vi "DMM User Interface.vi"() -> ()   [LabVIEW 2023, in "GUI.lvlib" / "Diagnostic.lvlib"]
uses:
  Diagnostic.lvlib
  <instrlib>/niDMM/nidmm.llb/niDMM Resolution in Digits.ctl
  <instrlib>/niDMM/nidmm.llb/niDMM Function.ctl
panel:
  in  "Stop":bool caption="Blank"
  in  "Apply":bool caption="Blank"
  in  "DMM Operation":T1(tab)
  in  "DMM":refnum<k15>="PXI2Slot6"
  out "Measured Value":dbl=1e-06 caption="Absolute Resolution (1E-6)" format="%.4f"
  in  "Range":dbl=-1.0
  in  "Resolution in Digits":T2=5.5 items=["3 1/2"=3.5, "4 1/2"=4.5, "5 1/2"=5.5, "6 1/2"=6.5, "7 1/2"=7.5]
  in  "Measurement Function (DC Volts)":T3=enum."Diode" caption="Measurement Function"
  # "Digital MultiMeter"
  # "Operation:"
  # "Self Test is Enabled by selecting\n            this opeartion"
  # "DMM Close Operation will be executing \nby selecting this opeartion"
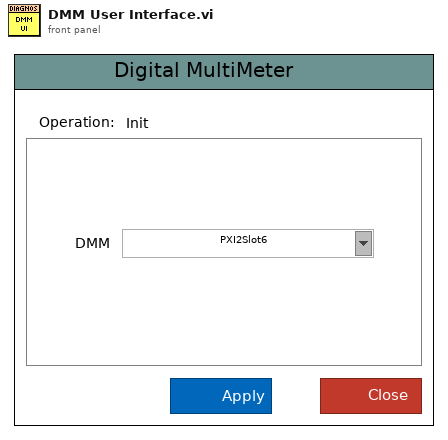
[diagram p1: front panel]
types:
  T1 = enum32{"Init", "Self Test", "Configure", "Measure", "Generate", "Close"}
  T2 = typedef "niDMM Resolution in Digits.ctl" = dbl
  T3 = typedef "niDMM Function.ctl" = enum16{"DC Volts", "AC Volts", "DC Current", "AC Current", "2-wire Resistance", "4-wire Resistance", "Diode", "Frequency", "Period", "AC Volts DC Coupled", "Capacitance", "Inductance", "Temperature"}
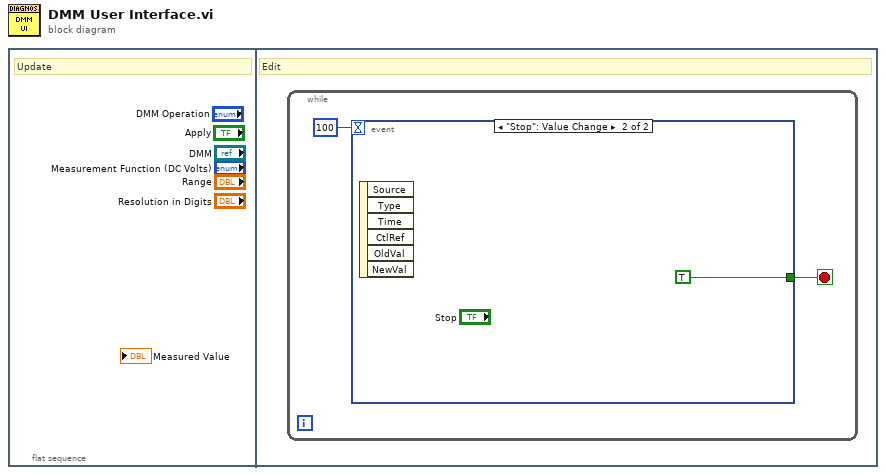
[diagram p0: block diagram]
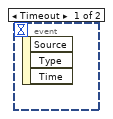
[diagram p2: hidden frame]
diagram:
  n1 = flat-sequence {
    frame #0 {
      # "Update"
    }
    frame #1 {
      # "Edit"
      n2 = while {
        stop <- w1 stop-if-true
        n3 = event shown="[1] \"Stop\": Value Change" {
          selector: _ -> [_ _]
          dyn-events: _ -> [_ _]
          timeout: 100 -> [_ _]
          tunnel: [_ TRUE] -> w1
          event Timeout {
            n4 = event-data() -> ()  [unwired: 1 in, 3 out]
          }
          event "Stop": Value Change {
            n5 = event-data() -> ()  [unwired: 1 in, 6 out]
          }
        }
      }
    }
  }
